vi "Finalize Settings 1.0.vi"(8 "error in (no error)":errorcluster, 11 "configuration 1.0":cluster{"name":string}={"name"="Transfer"}) -> (0 "error out":errorcluster, 2 "settings version":T1, 3 "settings 1.0":cluster{"key":string, "value":string}[](array[cluster]))   [LabVIEW 2017, in "DSF Core.lvlib" / "Core Transfer Configuration.lvclass"]
uses:
  Core Transfer Configuration.lvclass
  Typedefs/DSF Version Info.ctl
  DSF Core.lvlib
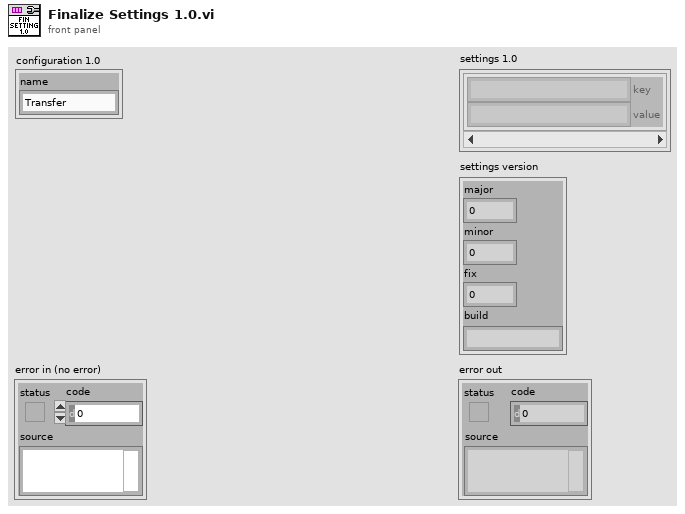
[diagram p1: front panel]
types:
  T1 = typedef "DSF Core.lvlib/DSF Version Info.ctl" = cluster{"major":u32, "minor":u32, "fix":u32, "build":string}
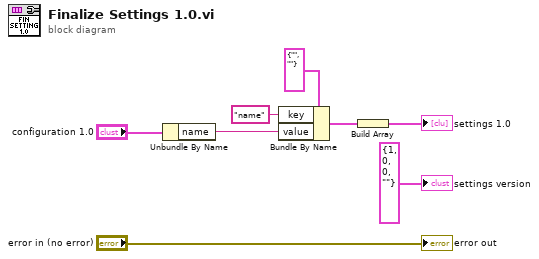
[diagram p0: block diagram]
diagram:
  n1 = Unbundle By Name("configuration 1.0") -> ("name"=w5:string)
  n2 = Bundle By Name(cluster=cluster{"key":string, "value":string} {"key"="", "value"=""} ("setting"), "key"="name", "value"=w5) -> (w3:cluster{"key":string, "value":string})
  n3 = Build Array(w3) -> (→"settings 1.0":cluster{"key":string, "value":string}[])
  "error out" <- "error in (no error)"
  "settings version" <- T1 {"major"=1, "minor"=0, "fix"=0, "build"=""} ("settings version")
